vi "PS-RA06B FPGA.vi"() -> ()   [LabVIEW 2011]
uses:
  <vilib>/rvi/eio/common/nirviEmuTemplateMethod_errors.vi
  <vilib>/eio/EIONode/EIONode.xnode
  <vilib>/rvi/Analysis/measure/butterworth/XNode/niFpgaButterworthFilter.xnode
  <vilib>/eio/EIOMethodNode/EIOMethodNode.xnode
panel:
  out "Mod5/AI2":fxp<+/-,20,5> format="%.17g"
  out "Mod5/AI0":fxp<+/-,20,5> format="%.17g"
  out "Mod5/AI1":fxp<+/-,20,5> format="%.17g"
  out "Mod1/AI2":fxp<+/-,20,5> format="%.17g"
  out "Mod1/AI3":fxp<+/-,20,5> format="%.17g"
  out "Mod1/AI0":fxp<+/-,20,5> format="%.17g"
  out "Mod1/AI1":fxp<+/-,20,5> format="%.17g"
  out "Mod5/AI3":fxp<+/-,20,5> format="%.17g"
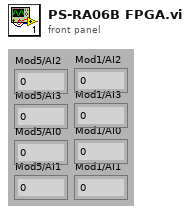
[diagram p1: front panel]
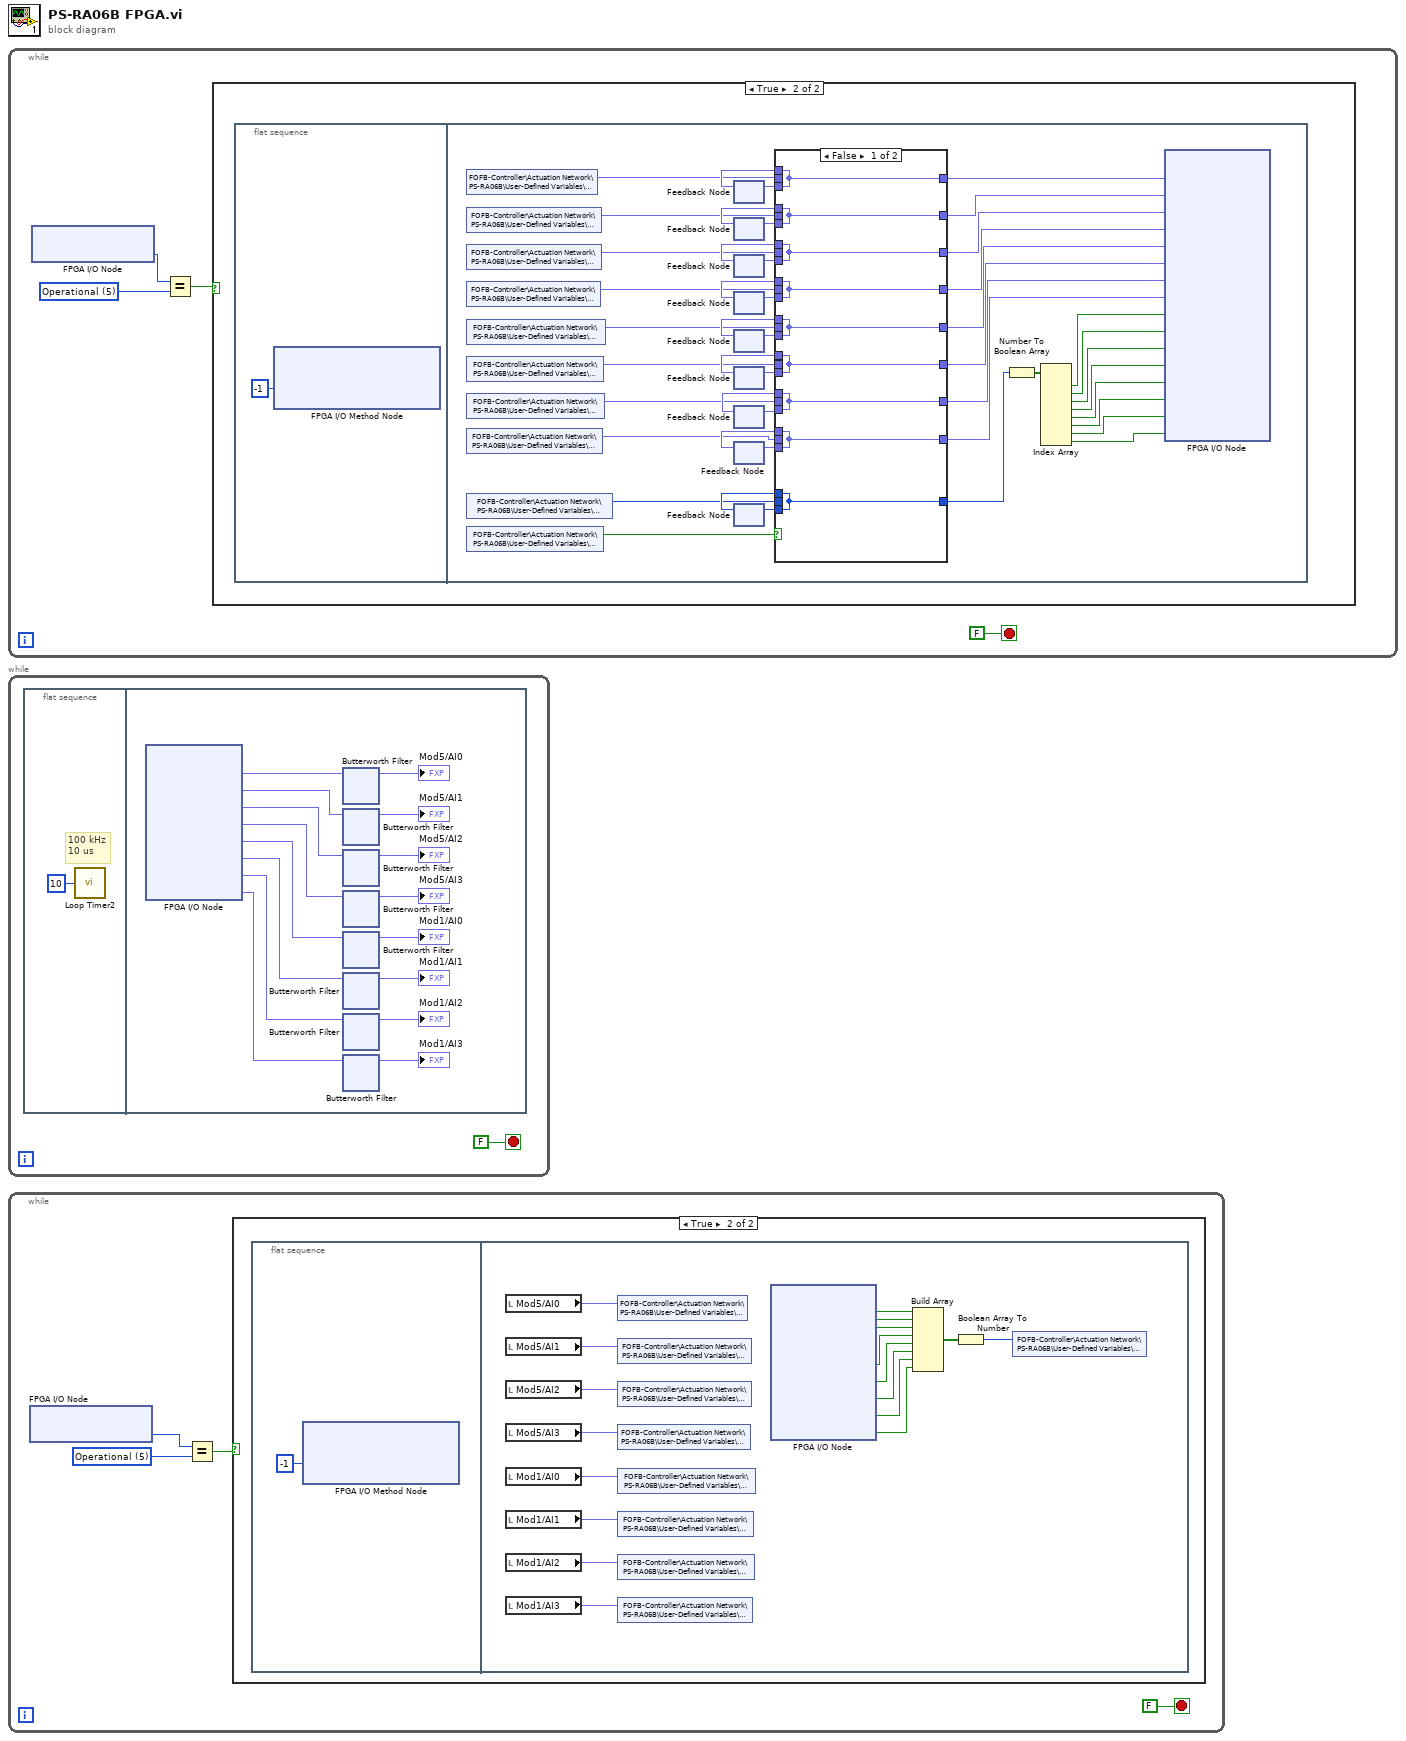
[diagram p0: block diagram]
diagram:
  n1 = while {
    stop <- FALSE stop-if-true
    w1 = u8 5 items=["Init"=1, "PreOp"=2, "Bootstrap"=3, "SafeOp"=4, "Operational"=5]
    n2 = xnode "FPGA I/O Node"() -> ("EtherCAT State"=w2:u8)  [unwired: 1 in, 1 out]
    n3 = Equal?(x=w2, y=w1) -> (x = y?=w3:bool)
    n4 = case shown="True" w3 {
      frame False {
      }
      frame True {
        n5 = flat-sequence {
          frame #0 {
            n6 = xnode "FPGA I/O Method Node"("Timeout"=-1) -> ()  [unwired: 1 in, 2 out]
          }
          frame #1 {
            n7 = shared-variable "FOFB-Controller\\Actuation Network\\PS-RA06B\\User-Defined Variables\\ACH12-Setpoint"() -> (w15:fxp<+/-,20,5>)  [unwired: 1 in, 1 out]
            n8 = shared-variable "FOFB-Controller\\Actuation Network\\PS-RA06B\\User-Defined Variables\\RRA06B-Setpoint"() -> (w14:fxp<+/-,20,5>)  [unwired: 1 in, 1 out]
            n9 = shared-variable "FOFB-Controller\\Actuation Network\\PS-RA06B\\User-Defined Variables\\ALV12A-Setpoint"() -> (w13:fxp<+/-,20,5>)  [unwired: 1 in, 1 out]
            n10 = shared-variable "FOFB-Controller\\Actuation Network\\PS-RA06B\\User-Defined Variables\\ALV12B-Setpoint"() -> (w12:fxp<+/-,20,5>)  [unwired: 1 in, 1 out]
            n11 = shared-variable "FOFB-Controller\\Actuation Network\\PS-RA06B\\User-Defined Variables\\ACH01A-Setpoint"() -> (w11:fxp<+/-,20,5>)  [unwired: 1 in, 1 out]
            n12 = shared-variable "FOFB-Controller\\Actuation Network\\PS-RA06B\\User-Defined Variables\\ACV01A-Setpoint"() -> (w10:fxp<+/-,20,5>)  [unwired: 1 in, 1 out]
            n13 = shared-variable "FOFB-Controller\\Actuation Network\\PS-RA06B\\User-Defined Variables\\ACH11B-Setpoint"() -> (w9:fxp<+/-,20,5>)  [unwired: 1 in, 1 out]
            n14 = shared-variable "FOFB-Controller\\Actuation Network\\PS-RA06B\\User-Defined Variables\\ACV11B-Setpoint"() -> (w8:fxp<+/-,20,5>)  [unwired: 1 in, 1 out]
            n15 = shared-variable "FOFB-Controller\\Actuation Network\\PS-RA06B\\User-Defined Variables\\PS-RA06B-ON-OFF"() -> (w7:u8)  [unwired: 1 in, 1 out]
            n16 = shared-variable "FOFB-Controller\\Actuation Network\\PS-RA06B\\User-Defined Variables\\PS-RA06B-Enable"() -> (w6:bool)  [unwired: 1 in, 1 out]
            n17 = feedback #1() -> (w17:fxp<+/-,20,5>)  [unwired: 1 in]
            n18 = feedback #2() -> (w36:fxp<+/-,20,5>)  [unwired: 1 in]
            n19 = feedback #3() -> (w39:fxp<+/-,20,5>)  [unwired: 1 in]
            n20 = feedback #4() -> (w40:fxp<+/-,20,5>)  [unwired: 1 in]
            n21 = feedback #5() -> (w42:fxp<+/-,20,5>)  [unwired: 1 in]
            n22 = feedback #6() -> (w45:fxp<+/-,20,5>)  [unwired: 1 in]
            n23 = feedback #7() -> (w48:fxp<+/-,20,5>)  [unwired: 1 in]
            n24 = feedback #8() -> (w46:fxp<+/-,20,5>)  [unwired: 1 in]
            n25 = feedback #9() -> (w51:u8)  [unwired: 1 in]
            n26 = case shown="False" w6 {
              tunnel: w15 -> [_ w69]
              tunnel: w17 -> [w60 _]
              tunnel: [w60 w69] -> w19
              tunnel: [w59 w68] -> w20
              tunnel: [w52 w67] -> w21
              tunnel: [w58 w62] -> w22
              tunnel: [w53 w63] -> w23
              tunnel: [w57 w64] -> w24
              tunnel: [w56 w65] -> w25
              tunnel: [w55 w66] -> w34
              tunnel: [w54 w61] -> w16
              tunnel: [w60 w69] -> w35
              tunnel: w14 -> [_ w68]
              tunnel: w8 -> [_ w66]
              tunnel: w36 -> [w59 _]
              tunnel: [w59 w68] -> w37
              tunnel: w13 -> [_ w67]
              tunnel: [w52 w67] -> w38
              tunnel: w39 -> [w52 _]
              tunnel: w12 -> [_ w62]
              tunnel: [w58 w62] -> w41
              tunnel: w40 -> [w58 _]
              tunnel: w11 -> [_ w63]
              tunnel: w42 -> [w53 _]
              tunnel: [w53 w63] -> w43
              tunnel: w10 -> [_ w64]
              tunnel: [w57 w64] -> w44
              tunnel: w45 -> [w57 _]
              tunnel: w46 -> [w55 _]
              tunnel: [w55 w66] -> w47
              tunnel: w48 -> [w56 _]
              tunnel: [w56 w65] -> w49
              tunnel: w9 -> [_ w65]
              tunnel: [w54 w61] -> w50
              tunnel: w7 -> [_ w61]
              tunnel: w51 -> [w54 _]
              frame False {
              }
              frame True {
              }
            }
            n27 = feedback-in #1(w35) -> ()
            n28 = feedback-in #2(w37) -> ()
            n29 = feedback-in #3(w38) -> ()
            n30 = feedback-in #4(w41) -> ()
            n31 = feedback-in #5(w43) -> ()
            n32 = feedback-in #6(w44) -> ()
            n33 = feedback-in #7(w49) -> ()
            n34 = feedback-in #8(w47) -> ()
            n35 = feedback-in #9(w50) -> ()
            n36 = Number To Boolean Array(number=w16) -> (Boolean array=w18:bool[])
            n37 = Index Array(array=w18) -> (element #1=w26:bool, element #2=w27:bool, element #3=w28:bool, element #4=w29:bool, element #5=w33:bool, element #6=w30:bool, element #7=w31:bool, element #8=w32:bool)  [unwired: 8 in]
            n38 = xnode "FPGA I/O Node"("Mod6/AO0"=w19, "Mod6/AO1"=w20, "Mod6/AO2"=w21, "Mod6/AO3"=w22, "Mod2/AO0"=w23, "Mod2/AO1"=w24, "Mod2/AO2"=w25, "Mod2/AO3"=w34, "Mod4/DIO6"=w26, "Mod4/DIO7"=w27, "Mod4/DIO4"=w28, "Mod4/DIO5"=w29, "Mod4/DIO2"=w33, "Mod4/DIO3"=w30, "Mod4/DIO0"=w31, "Mod4/DIO1"=w32) -> ()  [unwired: 16 in, 16 out]
          }
        }
      }
    }
  }
  n39 = while {
    stop <- FALSE stop-if-true
    n40 = flat-sequence {
      frame #0 {
        # "100 kHz\n10 us"
        n41 = call "Loop Timer2"("Count(uSec)"=u8 10) -> ()  [unwired: 1 out]
      }
      frame #1 {
        n42 = xnode "FPGA I/O Node"() -> ("Mod5/AI0"=w87:fxp<+/-,20,5>, "Mod5/AI1"=w86:fxp<+/-,20,5>, "Mod5/AI2"=w85:fxp<+/-,20,5>, "Mod5/AI3"=w84:fxp<+/-,20,5>, "Mod1/AI0"=w83:fxp<+/-,20,5>, "Mod1/AI1"=w82:fxp<+/-,20,5>, "Mod1/AI2"=w81:fxp<+/-,20,5>, "Mod1/AI3"=w80:fxp<+/-,20,5>)  [unwired: 8 in, 8 out]
        n43 = xnode "Butterworth Filter"("input data"=w87) -> ("output data"=→"Mod5/AI0":fxp<+/-,20,5>)  [unwired: 2 in]
        n44 = xnode "Butterworth Filter"("input data"=w86) -> ("output data"=→"Mod5/AI1":fxp<+/-,20,5>)  [unwired: 2 in]
        n45 = xnode "Butterworth Filter"("input data"=w85) -> ("output data"=→"Mod5/AI2":fxp<+/-,20,5>)  [unwired: 2 in]
        n46 = xnode "Butterworth Filter"("input data"=w84) -> ("output data"=→"Mod5/AI3":fxp<+/-,20,5>)  [unwired: 2 in]
        n47 = xnode "Butterworth Filter"("input data"=w83) -> ("output data"=→"Mod1/AI0":fxp<+/-,20,5>)  [unwired: 2 in]
        n48 = xnode "Butterworth Filter"("input data"=w82) -> ("output data"=→"Mod1/AI1":fxp<+/-,20,5>)  [unwired: 2 in]
        n49 = xnode "Butterworth Filter"("input data"=w81) -> ("output data"=→"Mod1/AI2":fxp<+/-,20,5>)  [unwired: 2 in]
        n50 = xnode "Butterworth Filter"("input data"=w80) -> ("output data"=→"Mod1/AI3":fxp<+/-,20,5>)  [unwired: 2 in]
      }
    }
  }
  n51 = while {
    stop <- FALSE stop-if-true
    w146 = u8 5 items=["Init"=1, "PreOp"=2, "Bootstrap"=3, "SafeOp"=4, "Operational"=5]
    n52 = xnode "FPGA I/O Node"() -> ("EtherCAT State"=w145:u8)  [unwired: 1 in, 1 out]
    n53 = Equal?(x=w145, y=w146) -> (x = y?=w144:bool)
    n54 = case shown="True" w144 {
      frame False {
      }
      frame True {
        n55 = flat-sequence {
          frame #0 {
            n56 = xnode "FPGA I/O Method Node"("Timeout"=-1) -> ()  [unwired: 1 in, 2 out]
          }
          frame #1 {
            n57 = local read "Mod5/AI0"() -> (w164:fxp<+/-,20,5>)
            n58 = local read "Mod5/AI1"() -> (w163:fxp<+/-,20,5>)
            n59 = local read "Mod5/AI2"() -> (w162:fxp<+/-,20,5>)
            n60 = local read "Mod5/AI3"() -> (w160:fxp<+/-,20,5>)
            n61 = local read "Mod1/AI0"() -> (w159:fxp<+/-,20,5>)
            n62 = local read "Mod1/AI1"() -> (w158:fxp<+/-,20,5>)
            n63 = local read "Mod1/AI2"() -> (w157:fxp<+/-,20,5>)
            n64 = local read "Mod1/AI3"() -> (w161:fxp<+/-,20,5>)
            n65 = shared-variable "FOFB-Controller\\Actuation Network\\PS-RA06B\\User-Defined Variables\\ACH12-Reading"(w164) -> ()  [unwired: 1 in, 1 out]
            n66 = shared-variable "FOFB-Controller\\Actuation Network\\PS-RA06B\\User-Defined Variables\\RRA06B-Reading"(w163) -> ()  [unwired: 1 in, 1 out]
            n67 = shared-variable "FOFB-Controller\\Actuation Network\\PS-RA06B\\User-Defined Variables\\ALV12A-Reading"(w162) -> ()  [unwired: 1 in, 1 out]
            n68 = shared-variable "FOFB-Controller\\Actuation Network\\PS-RA06B\\User-Defined Variables\\ALV12B-Reading"(w160) -> ()  [unwired: 1 in, 1 out]
            n69 = shared-variable "FOFB-Controller\\Actuation Network\\PS-RA06B\\User-Defined Variables\\ACH01A-Reading"(w159) -> ()  [unwired: 1 in, 1 out]
            n70 = shared-variable "FOFB-Controller\\Actuation Network\\PS-RA06B\\User-Defined Variables\\ACV01A-Reading"(w158) -> ()  [unwired: 1 in, 1 out]
            n71 = shared-variable "FOFB-Controller\\Actuation Network\\PS-RA06B\\User-Defined Variables\\ACH11B-Reading"(w157) -> ()  [unwired: 1 in, 1 out]
            n72 = shared-variable "FOFB-Controller\\Actuation Network\\PS-RA06B\\User-Defined Variables\\ACV11B-Reading"(w161) -> ()  [unwired: 1 in, 1 out]
            n73 = xnode "FPGA I/O Node"() -> ("Mod3/DIO6"=w156:bool, "Mod3/DIO7"=w155:bool, "Mod3/DIO4"=w154:bool, "Mod3/DIO5"=w153:bool, "Mod3/DIO2"=w152:bool, "Mod3/DIO3"=w151:bool, "Mod3/DIO0"=w150:bool, "Mod3/DIO1"=w149:bool)  [unwired: 8 in, 8 out]
            n74 = Build Array(w156, w155, w154, w153, w152, w151, w150, w149) -> (w166:bool[])
            n75 = Boolean Array To Number(Boolean array=w166) -> (number=w165:u8)
            n76 = shared-variable "FOFB-Controller\\Actuation Network\\PS-RA06B\\User-Defined Variables\\PS-RA06B-Status"(w165) -> ()  [unwired: 1 in, 1 out]
          }
        }
      }
    }
  }
